vi "remove_start_end_space.vi"(8 "error in (no error)":errorcluster, 11 "String":string="SA DFFSDFA   ") -> (0 "error out":errorcluster, 3 "after substring":string)   [LabVIEW 2018]
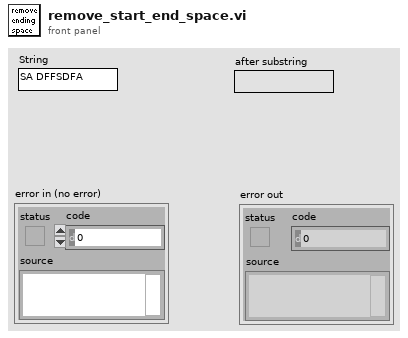
[diagram p1: front panel]
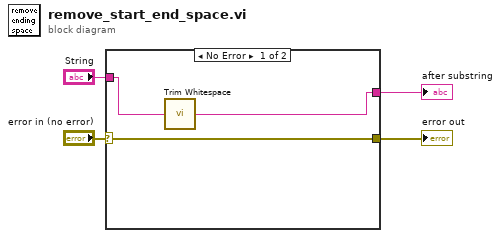
[diagram p0: block diagram]
diagram:
  n1 = case shown="No Error" "error in (no error)" {
    selector: "error in (no error)" -> [w7 w8]
    tunnel: "String" -> [w6 w9]
    tunnel: [w5 w9] -> w3
    tunnel: [w7 w8] -> w1
    frame No Error {
      n2 = call <vilib>:"Trim Whitespace.vi"("string"=w6) -> ("trimmed string"=w5:string)  [unwired: 1 in]
    }
    frame Error {
    }
  }
  "after substring" <- w3
  "error out" <- w1
